vi "New motor Control integrated, PID based accel.vi"(3 "xTargetSpeed":dbl, 4 "yTargetSpeed":dbl, 5 "wTargetSpeed":dbl) -> ()   [LabVIEW 2018]
uses:
  <vilib>/addons/control/pid/pid.llb/PID (DBL).vi
  <vilib>/addons/control/pid/NI_PID_pid.lvlib
panel:
  out "yTargetSpeed 2":dbl
  out "ySpeed":dbl
  out "Waveform Chart":dynamicdata(graph)
  out "Numeric 3":dbl
  out "Numeric 2":dbl
  out "Numeric":dbl
  out "Speed":T1
  out "Distance M2":dbl
  out "Distance M1":dbl
  out "Distance M0":dbl
  in  "Boolean":bool=TRUE
  out "Motor Error":errorcluster
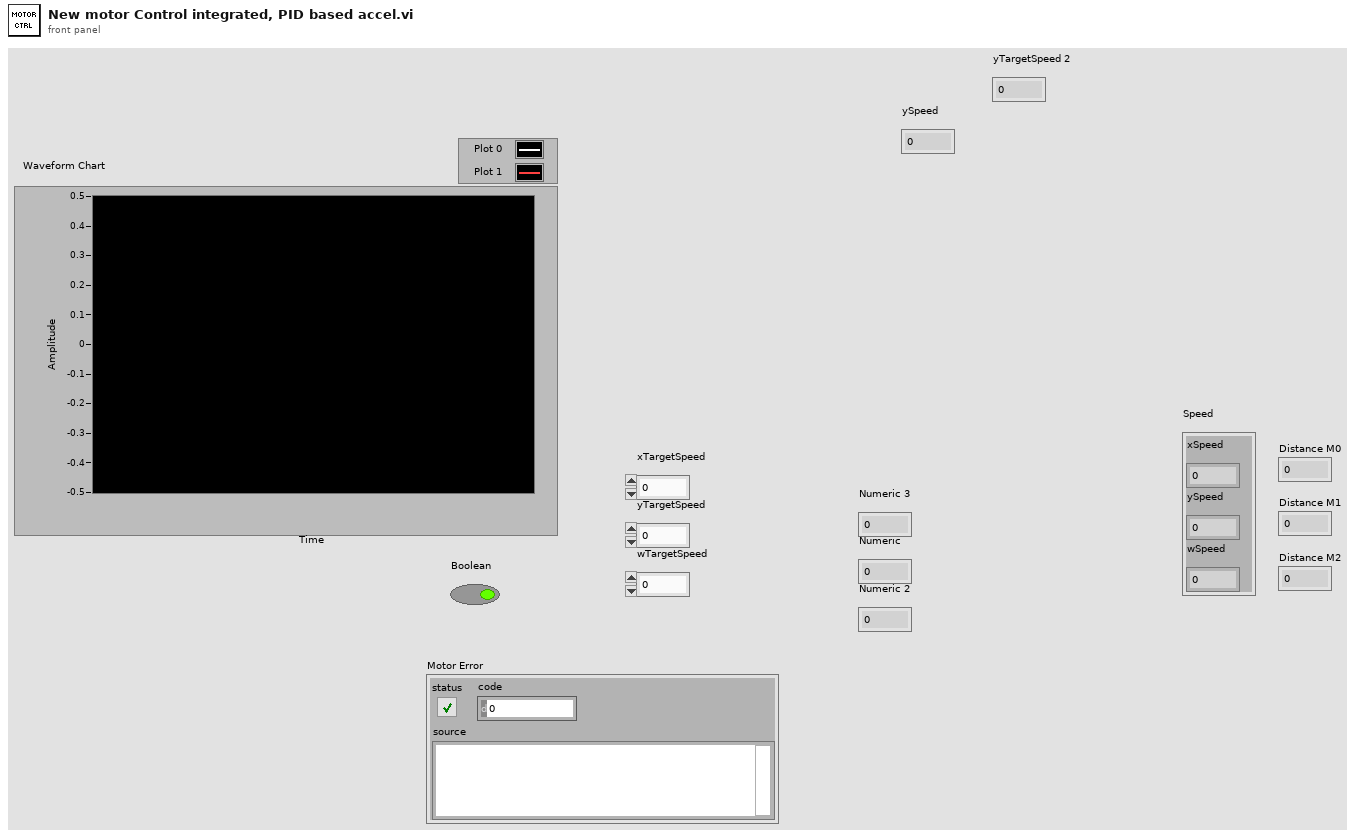
[diagram p1: front panel]
types:
  T1 = cluster{"xSpeed":dbl, "ySpeed":dbl, "wSpeed":dbl}
  T2 = cluster{"Encoder 0":dbl, "Encoder 1":dbl, "Encoder 2":dbl}
  T3 = cluster{"proportional gain (Kc)":dbl, "integral time (Ti, min)":dbl, "derivative time (Td, min)":dbl}
  T4 = cluster{"Distance M0 ":dbl, "Distance M1 ":dbl, "Distance M2 ":dbl}
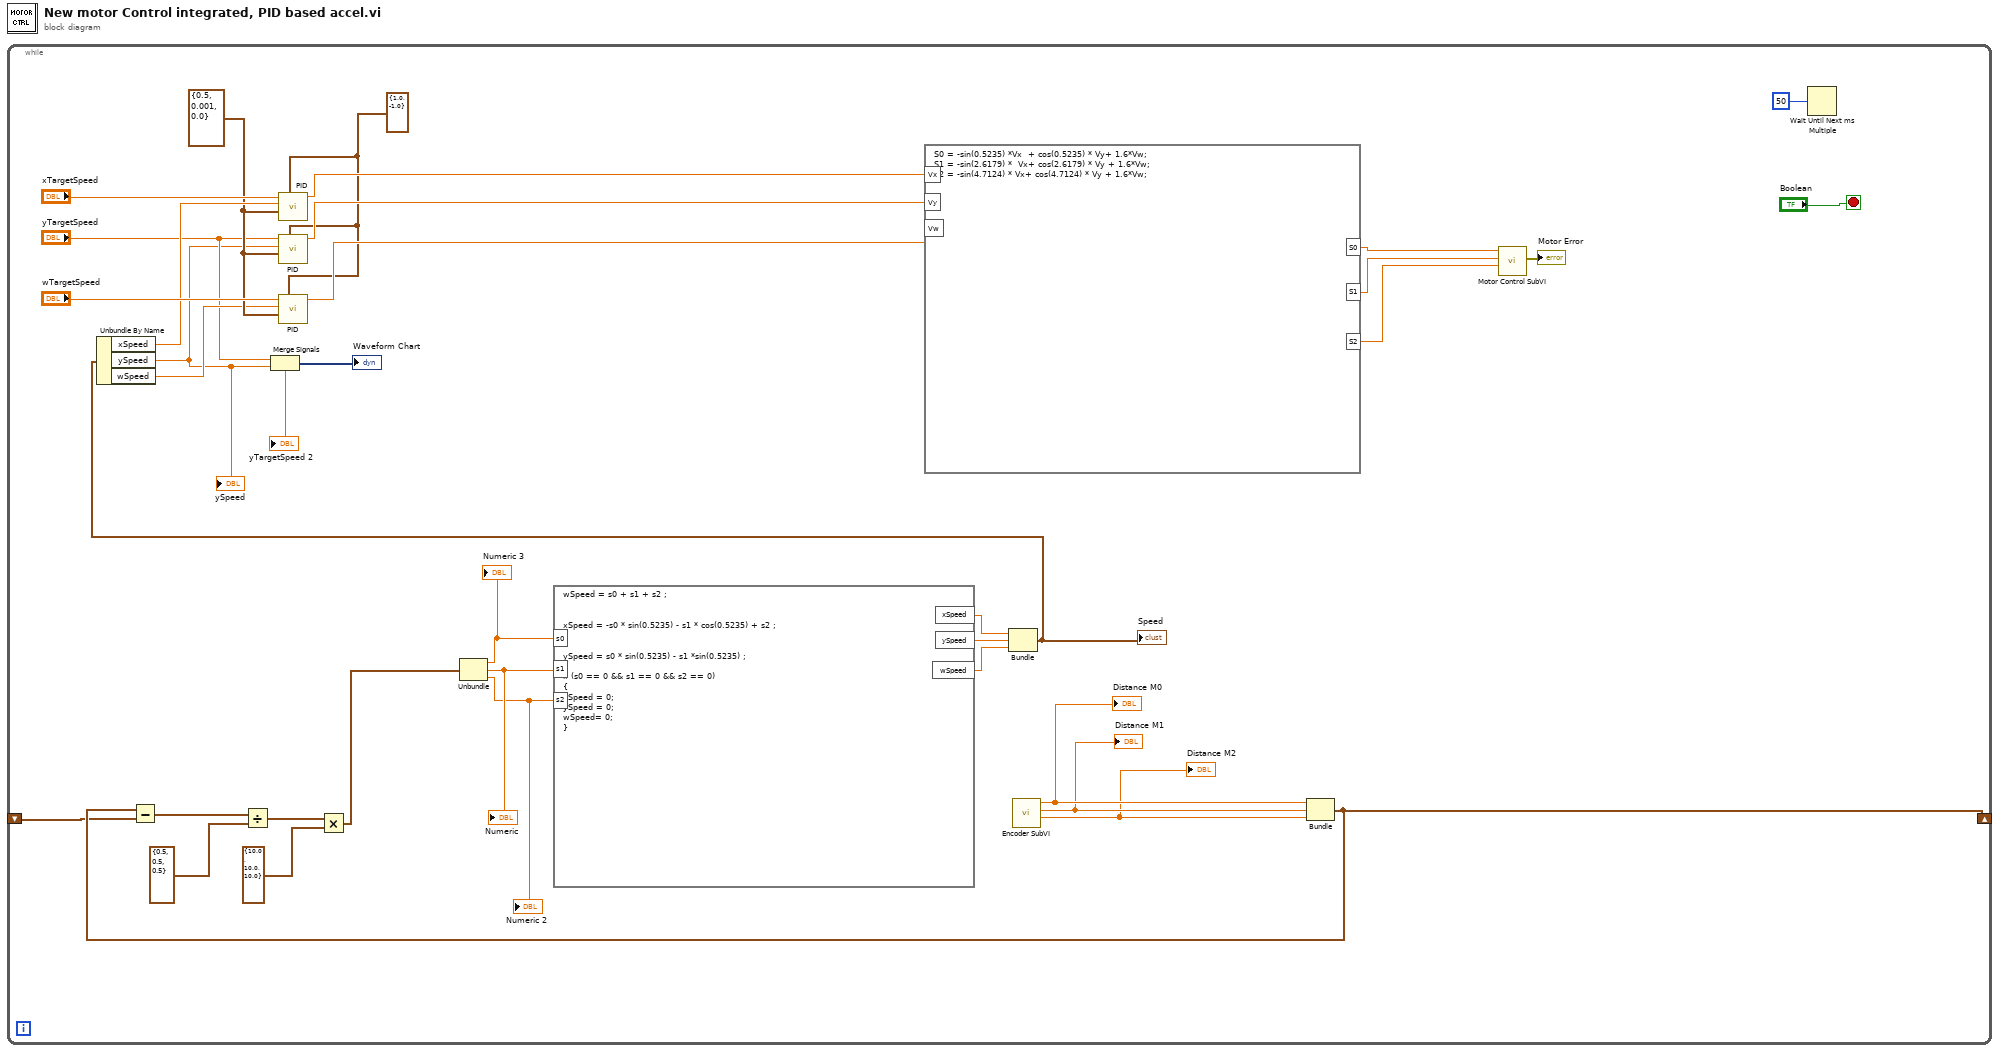
[diagram p0: block diagram]
diagram:
  n1 = while {
    shift-right: [w2] -> _
    shift-left: _ -> [w1]
    stop <- "Boolean" stop-if-true
    w7 = cluster{"output high":dbl, "output low":dbl} {"output high"=1.0, "output low"=-1.0} ("output range")
    w10 = T3 {"proportional gain (Kc)"=0.5, "integral time (Ti, min)"=0.001, "derivative time (Td, min)"=0.0} ("PID gains")
    n2 = call "Encoder SubVI.vi"() -> ("Distance M2"=w24:dbl, "Distance M1"=w25:dbl, "Distance M0"=w26:dbl)  [unwired: 8 in, 1 out]
    "Distance M0" <- w26
    "Distance M1" <- w25
    "Distance M2" <- w24
    n3 = Bundle("Distance M0"=w26, "Distance M1"=w25, "Distance M2"=w24) -> (w2:T4)  [unwired: 1 in]
    n4 = Subtract(x=w2, y=w1) -> (x-y=w34:T4)
    n5 = Divide(x=w34, y=T2 {"Encoder 0"=0.5, "Encoder 1"=0.5, "Encoder 2"=0.5}) -> (x/y=w20:cluster{dbl, dbl, dbl})
    n6 = Multiply(x=w20, y=cluster{dbl, dbl, dbl} {10.0, 10.0, 10.0}) -> (x*y=w18:cluster{dbl, dbl, dbl})
    n7 = Unbundle(w18) -> (w17:dbl, w16:dbl, w15:dbl)
    "Numeric" <- w16
    "Numeric 2" <- w15
    "Numeric 3" <- w17
    n8 = formula code="wSpeed = s0 + s1 + s2 ;\n\n\nxSpeed = -s0 * sin(0.5235) - s1 * cos(0.5235) + s2 ;\n\n\nySpeed = s0 * sin(0.5235) - s1 *sin(0.5235) ;\n\nif (s0 == 0 && s1 == 0 && s2 == 0)\n{\nxSpeed = 0;\nySpeed = 0;\nwSpeed= 0;\n}"("s0"=w17, "s1"=w16, "s2"=w15) -> ("xSpeed"=w31:dbl, "ySpeed"=w32:dbl, "wSpeed"=w30:dbl)
    n9 = Bundle("xSpeed"=w31, "ySpeed"=w32, "wSpeed"=w30) -> (w29:T1)  [unwired: 1 in]
    "Speed" <- w29
    n10 = Unbundle By Name(w29) -> ("xSpeed"=w11:dbl, "ySpeed"=w4:dbl, "wSpeed"=w6:dbl)
    "ySpeed" <- w4
    n11 = Merge Signals("yTargetSpeed", w4) -> (→"Waveform Chart":dynamicdata)
    n12 = call-poly <vilib>:"PID.vi"("output range"=w7, "PID gains"=w10, "process variable"=w11, "setpoint"="xTargetSpeed") -> ("output"=w13:dbl)  [unwired: 6 in, 1 out]
    n13 = call-poly <vilib>:"PID.vi"("output range"=w7, "PID gains"=w10, "process variable"=w4, "setpoint"="yTargetSpeed") -> ("output"=w9:dbl)  [unwired: 6 in, 1 out]
    n14 = call-poly <vilib>:"PID.vi"("output range"=w7, "PID gains"=w10, "process variable"=w6, "setpoint"="wTargetSpeed") -> ("output"=w8:dbl)  [unwired: 6 in, 1 out]
    n15 = formula code="S0 = -sin(0.5235) *Vx  + cos(0.5235) * Vy+ 1.6*Vw;\nS1 = -sin(2.6179) *  Vx+ cos(2.6179) * Vy + 1.6*Vw;\nS2 = -sin(4.7124) * Vx+ cos(4.7124) * Vy + 1.6*Vw;"("Vx"=w13, "Vy"=w9, "Vw"=w8) -> ("S0"=w23:dbl, "S1"=w22:dbl, "S2"=w21:dbl)
    n16 = call "Motor Control SubVI.vi"("Speed M2"=w21, "Speed M1"=w22, "Speed M0"=w23) -> ("Motor Error"=→"Motor Error":errorcluster)  [unwired: 8 in]
    n17 = Wait Until Next ms Multiple(millisecond multiple=u32 50) -> ()  [unwired: 1 out]
    "yTargetSpeed 2" <- "yTargetSpeed"
  }
